vi "Launch Heater Actor.vi"(4 "PID.":T3={"PID"={"P"=10.0, "I"=1.5, "D"=5.0}, "Upper Limit"=100.0, "Lower Limit"=-100.0}, 5 "DedicatedEnQrs":refnum<queue>, 6 "SHVs":T2, 7 "Name":string="Heater", 8 "error in (no error)":errorcluster, 9 "Freezer":T1, 10 "Interlock Chain":refnum<class "Interlock Chain.lvclass">, 11 "Caller Actor in":refnum<class "Actor.lvclass">) -> (0 "error out":errorcluster, 3 "Caller-To-Actor Enqueuer":refnum<class "Message Enqueuer.lvclass">)   [LabVIEW 2015, in "cRIO-Carbondioxide.lvlib" / "CO2-Actor.lvlib" / "Heater.lvclass"]
uses:
  Heater.lvclass
  <vilib>/ActorFramework/Message Enqueuer/Message Enqueuer.lvclass
  <vilib>/ActorFramework/Actor/Actor.lvclass
  Interlocks/Interlock Chain/Interlock Chain.lvclass
  cRIO-CO2/Freezers Enumerator.ctl
  Controls/Dedicated Enqueuers.ctl
  CO2 Actor/CO2 Actor.lvclass
  Heater.lvclass/Heater.ctl
  cRIO-CO2/cRIO-CO2.lvclass
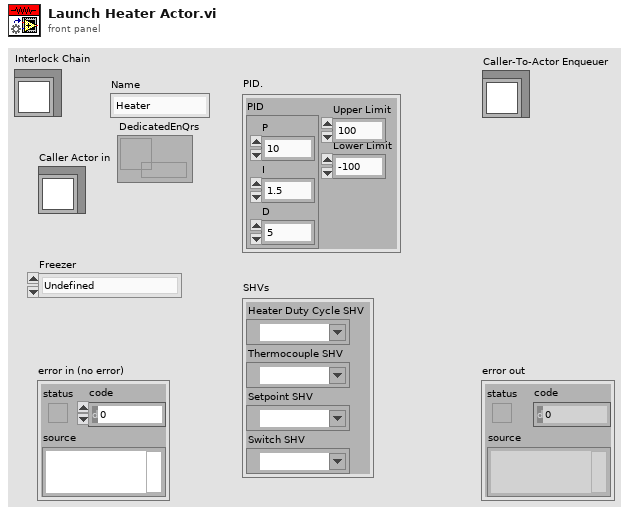
[diagram p1: front panel]
types:
  T1 = typedef "cRIO-Carbondioxide.lvlib/cRIO-CO2.lvlib/cRIO-CO2.lvclass/Freezers Enumerator.ctl" = enum16{"Undefined", "Syringe", "Cold Tank 1", "Cold Tank 2", "Cold Tank 3", "Cold Tank 4"}
  T2 = cluster{"Heater Duty Cycle SHV":refnum<k21>, "Thermocouple SHV":refnum<k21>, "Setpoint SHV":refnum<k21>, "Switch SHV":refnum<k21>}
  T3 = cluster{"PID":cluster{"P":dbl, "I":dbl, "D":dbl}, "Upper Limit":dbl, "Lower Limit":dbl}
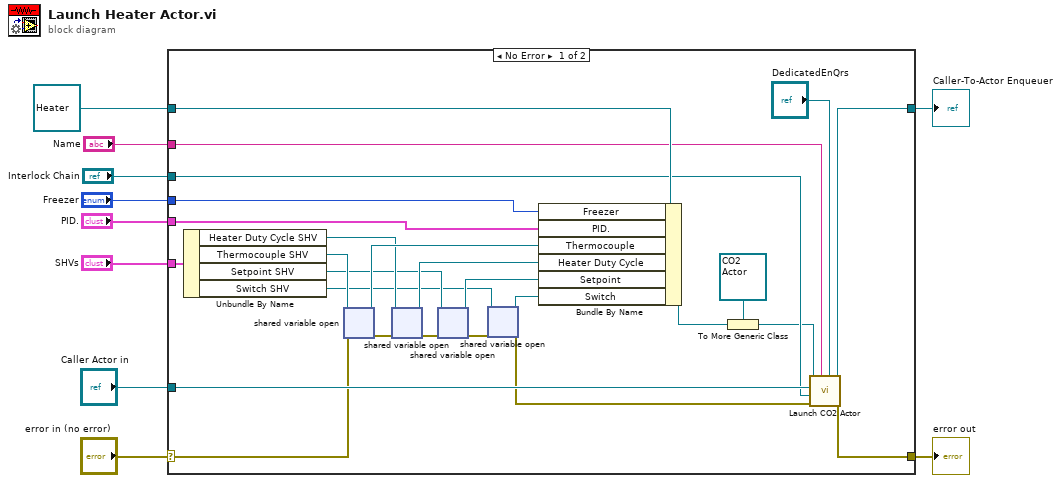
[diagram p0: block diagram]
diagram:
  n1 = case shown="No Error" "error in (no error)" {
    selector: "error in (no error)" -> [w30 w37]
    tunnel: [w35 w37] -> w9
    tunnel: [w36 _] -> w7
    tunnel: refnum<class "Heater.lvclass"> refnum ("Heater in") -> [w18 _]
    tunnel: "Name" -> [w17 _]
    tunnel: "Caller Actor in" -> [w34 _]
    tunnel: "PID." -> [w29 _]
    tunnel: "Interlock Chain" -> [w16 _]
    tunnel: "SHVs" -> [w19 _]
    tunnel: "Freezer" -> [w12 _]
    frame No Error {
      n2 = Unbundle By Name(w19) -> ("Heater Duty Cycle SHV"=w23:refnum<k21>, "Thermocouple SHV"=w22:refnum<k21>, "Setpoint SHV"=w21:refnum<k21>, "Switch SHV"=w20:refnum<k21>)
      n3 = shared-variable-open(w22, w30) -> (w33:refnum<k21>, w32:errorcluster)
      n4 = shared-variable-open(w23, w32) -> (w31:refnum<k21>, w28:errorcluster)
      n5 = shared-variable-open(w21, w28) -> (w27:refnum<k21>, w26:errorcluster)
      n6 = shared-variable-open(w20, w26) -> (w24:refnum<k21>, w25:errorcluster)
      n7 = Bundle By Name(cluster=w18, "Freezer"=w12, "PID."=w29, "Thermocouple"=w33, "Heater Duty Cycle"=w31, "Setpoint"=w27, "Switch"=w24) -> (w14:refnum<class "Heater.lvclass">)
      n8 = To More Generic Class(target class=refnum<class "CO2 Actor.lvclass"> refnum ("CO2 Actor in"), reference=w14) -> (generic class reference=w13:refnum<class "CO2 Actor.lvclass">)
      n9 = call "Launch CO2 Actor.vi"("DedicatedEnQrs"="DedicatedEnQrs", "Name"=w17, "error in (no error)"=w25, "Interlock Chain"=w16, "Caller Actor in"=w34, "CO2 Actor in"=w13) -> ("error out"=w35:errorcluster, "Caller-To-Actor Enqueuer"=w36:refnum<class "Message Enqueuer.lvclass">)  [unwired: 4 in]
    }
    frame Error {
    }
  }
  "error out" <- w9
  "Caller-To-Actor Enqueuer" <- w7
